vi "Smart Open With Range.vi"(4 "Max Value":dbl[](array[numeric]), 6 "Min Value":dbl[](array[numeric]), 7 "Allow multiple opens?":bool=TRUE, 8 "error in (no error)":errorcluster, 10 "Channel Names":tag[](array[tag])) -> (0 "error out":errorcluster, 3 "AI Ref Out":T1)   [LabVIEW 2021, in "AI.lvlib"]
uses:
  <vilib>/myRIO/Instrument Drivers/Onboard IO/AI/AI.lvlib
  <vilib>/myRIO/Instrument Drivers/Onboard IO/AI/vis/myRIO AI Open.xnode
  <vilib>/myRIO/Common/Instrument Driver Framework/Utilities/typedefs/Analog Scaling Constants.ctl
  <vilib>/myRIO/Common/Instrument Driver Framework/Utilities/typedefs/Analog Scaling Constants List.ctl
  <vilib>/myRIO/Common/Instrument Driver Framework/myRIO v1.0/AI/typedefs/AI Channels Enum.ctl
  <vilib>/myRIO/Common/Instrument Driver Framework/myRIO v1.0/AI/typedefs/AI Channels List.ctl
  <vilib>/myRIO/Common/Instrument Driver Framework/Utilities/typedefs/Generic FPGA Reference.ctl
  <vilib>/myRIO/Common/Instrument Driver Framework/Utilities/typedefs/myRIO v1.0 Reference.ctl
  <vilib>/myRIO/Common/Instrument Driver Framework/Utilities/typedefs/Hardware Version Enum.ctl
  <vilib>/myRIO/Common/Instrument Driver Framework/Utilities/typedefs/myRIO Generic Hardware Reference.ctl
  <vilib>/myRIO/Instrument Drivers/Onboard IO/AI/typedefs/AI Reference.ctl
  <vilib>/myRIO/Common/Instrument Driver Framework/ELVIS III v1.0/AI/vis/ELVIS III v1.1 Open AI.vi
  <vilib>/userdefined/High Color/nirio_resource_hc.ctl
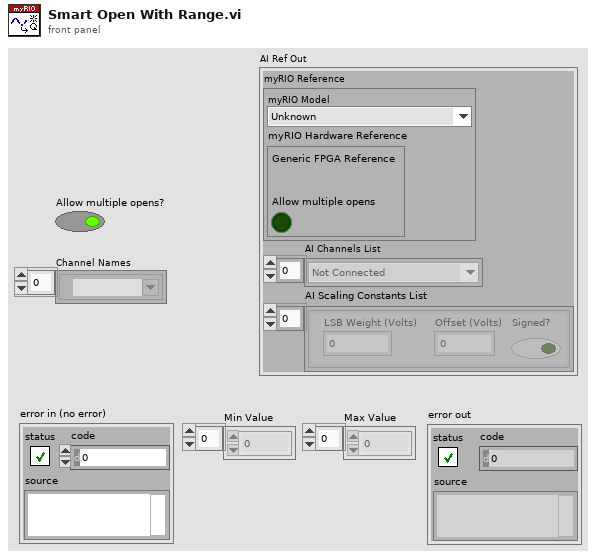
[diagram p1: front panel]
types:
  T1 = typedef "AI.lvlib/AI Reference.ctl" = cluster{"myRIO Reference":T2, "AI Channels List":T6, "AI Scaling Constants List":T8}
  T2 = typedef "myRIO Generic Hardware Reference.ctl" = cluster{"myRIO Model":T3, "myRIO Hardware Reference":T4}
  T3 = typedef "Hardware Version Enum.ctl" = enum16{"Unknown", "myRIO-1900", "myRIO-1950", "roboRIO", "NI ELVIS RIO CM", "ELVIS III"}
  T4 = typedef "myRIO v1.0 Reference.ctl" = cluster{"Generic FPGA Reference":T5, "Allow multiple opens":bool}
  T5 = typedef "Generic FPGA Reference.ctl" = refnum<k20>
  T6 = typedef "AI Channels List.ctl" = T7[]
  T7 = typedef "AI Channels Enum.ctl" = enum16{"Not Connected", "AudioIn/Left", "AudioIn/Right", "C/AI0", "C/AI1", "A/AI0", "A/AI1", "A/AI2", "A/AI3", "A/AI4", "A/AI5", "A/AI6", "A/AI7", "B/AI0", "B/AI1", "B/AI2", "B/AI3", "B/AI4", "B/AI5", "B/AI6", "B/AI7", "AI/AI0", "AI/AI1", "AI/AI2", "AI/AI3", "A/AI0 (DIFF)", "A/AI1 (DIFF)", "A/AI2 (DIFF)", "A/AI3 (DIFF)", "B/AI0 (DIFF)", "B/AI1 (DIFF)", "B/AI2 (DIFF)", "B/AI3 (DIFF)"}
  T8 = typedef "Analog Scaling Constants List.ctl" = T9[]
  T9 = typedef "Analog Scaling Constants.ctl" = cluster{"LSB Weight (Volts)":dbl, "Offset (Volts)":dbl, "Signed?":bool}
  T10 = typedef "nirio_resource_hc.ctl" = tag
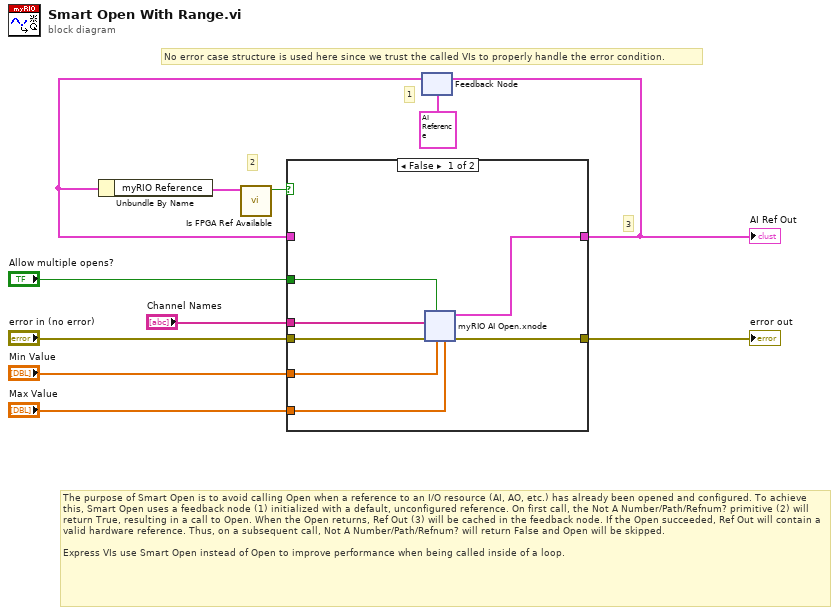
[diagram p0: block diagram]
diagram:
  # "No error case structure is used here since we trust the called VIs to properly handle the error condition."
  # "3"
  # "1"
  # "2"
  # "The purpose of Smart Open is to avoid calling Open when a reference to an I/O resource (AI, AO, etc.) has already been opened and configured. To achieve this, Smart Open uses a feedback node (1) initialized with a default, unconfigured reference. On first call, the Not A Number/Path/Refnum? primitive (2) will return True, resulting in a call to Open. When the Open returns, Ref Out (3) will be cached in the feedback node. If the Open succeeded, Ref Out will contain a valid hardware reference. Thus, on a subsequent call, Not A Number/Path/Refnum? will return False and Open will be skipped.\n\t\nExpress VIs use Smart Open instead of Open to improve performance when being called inside of a loop."
  n1 = feedback #1(T1 {"myRIO Reference"={"myRIO Model"=enum."Unknown", "myRIO Hardware Reference"={"Generic FPGA Reference"=refnum, "Allow multiple opens"=FALSE}}, "AI Channels List"=[], "AI Scaling Constants List"=[]} ("AI Ref Out")) -> (w6:T1)
  n2 = Unbundle By Name(w6) -> ("myRIO Reference"=w3:T2)
  n3 = call <vilib>:"Is FPGA Ref Available.vi"("myRIO Reference"=w3) -> ("Is Available?"=w7:bool)  [unwired: 10 in]
  n4 = case shown="False" w7 {
    tunnel: "error in (no error)" -> [w18 w39]
    tunnel: [w17 w40] -> w9
    tunnel: [w16 w39] -> w10
    tunnel: w6 -> [_ w40]
    tunnel: "Allow multiple opens?" -> [w15 _]
    tunnel: "Channel Names" -> [w14 _]
    tunnel: "Min Value" -> [w13 _]
    tunnel: "Max Value" -> [w12 _]
    frame False {
      n5 = xnode "myRIO AI Open.xnode"("error in (no error)"=w18, "Allow multiple opens?"=w15, "Channel Names"=w14, "Max Value"=w12, "Min Value"=w13) -> ("error out"=w16:errorcluster, "AI Ref Out"=w17:T1)
    }
    frame True {
    }
  }
  "AI Ref Out" <- w9
  "error out" <- w10
  n6 = feedback-in #1(w9) -> ()
